vi "SubSpecOneCase.vi"(0 "Row":i32, 1 "Column":i32, 2 "Raw Fit Data":T1 {"pts in fit" format="%.2f"; "midband fit" format="%.2f"; "intercept (b)" format="%.2f"; "slope (m)" format="%.2f"}, 3 "Cal params":T2 {"pts in fit" format="%.2f"; "midband fit" format="%.2f"; "intercept (b)" format="%.2f"; "slope (m)" format="%.2f"}) -> (6 "single case fit data":T2 {"pts in fit" format="%.2f"; "midband fit" format="%.2f"; "intercept (b)" format="%.2f"; "slope (m)" format="%.2f"})   [LabVIEW 2022 SP3]
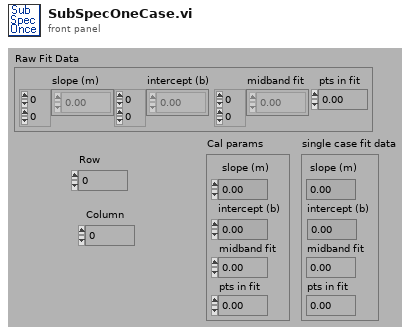
[diagram p1: front panel]
types:
  T1 = cluster{"slope (m)":dbl[][], "intercept (b)":dbl[][], "midband fit":dbl[][], "pts in fit":dbl}
  T2 = cluster{"slope (m)":dbl, "intercept (b)":dbl, "midband fit":dbl, "pts in fit":dbl}
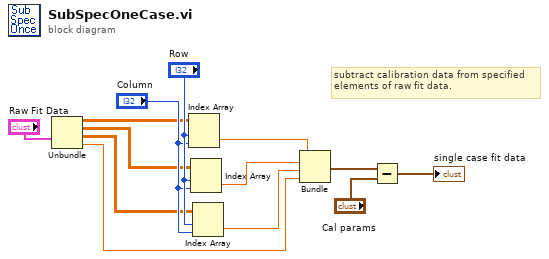
[diagram p0: block diagram]
diagram:
  # "subtract calibration data from specified\nelements of raw fit data."
  n1 = Unbundle("Raw Fit Data") -> ("slope (m)"=w7:dbl[][], "intercept (b)"=w4:dbl[][], "midband fit"=w2:dbl[][], "pts in fit"=w3:dbl)
  n2 = Index Array(array=w7, index (row)="Row", index (col)="Column") -> (element=w11:dbl)
  n3 = Index Array(array=w4, index (row)="Row", index (col)="Column") -> (element=w10:dbl)
  n4 = Index Array(array=w2, index (row)="Row", index (col)="Column") -> (element=w9:dbl)
  n5 = Bundle("slope (m)"=w11, "intercept (b)"=w10, "midband fit"=w9, "pts in fit"=w3) -> (w5:T2)  [unwired: 1 out]
  n6 = Subtract(x=w5, y="Cal params") -> (x-y=→"single case fit data":T2)
